vi "Launch.vi"(5 "Sequencer":refnum<class "MessageQ.lvclass">, 6 "State Control":T1, 7 "VolatusAPI":refnum<class "VolatusAPI.lvclass">, 8 "error in (no error)":refnum<class "MultiErrors.lvclass">, 10 "State":T2, 11 "State in":refnum<class "State.lvclass">) -> (0 "error out":refnum<class "MultiErrors.lvclass">, 3 "State out":refnum<class "State.lvclass">)   [LabVIEW 2023, in "VolatusSeq.lvlib" / "State.lvclass"]
uses:
  State.lvclass
  VolatusErrorUtilities/MultiErrors/MultiErrors.lvclass
  VolatusSeqConfig/State.ctl
  VolatusSeqConfig/Step.ctl
  VolatusSeqConfig/Command Config/Command Config.lvclass
  VolatusSeqConfig/Transition Config/Transition Config.lvclass
  VolatusSeqConfig/Debug Flags.ctl
  Volatus/VolatusAPI/VolatusAPI.lvclass
  State Control.ctl
  Sequence Time.ctl
  Variables/Variables.lvclass
  Volatus/MessageQ/MessageQ.lvclass
  lv-promises/Promises/Value/Value.lvclass
  lv-promises/Promises/Promise/Promise.lvclass/Promise.ctl
  lv-promises/Promises/Future/Future.lvclass/Future.ctl
  Loop Async.vi
  lv-promises/Promises/Future/Future.lvclass
  lv-promises/Promises/Promise/Promise.lvclass
  VolatusSeqConfig/VolatusSeqConfig.lvlib
  VolatusSeq.lvlib
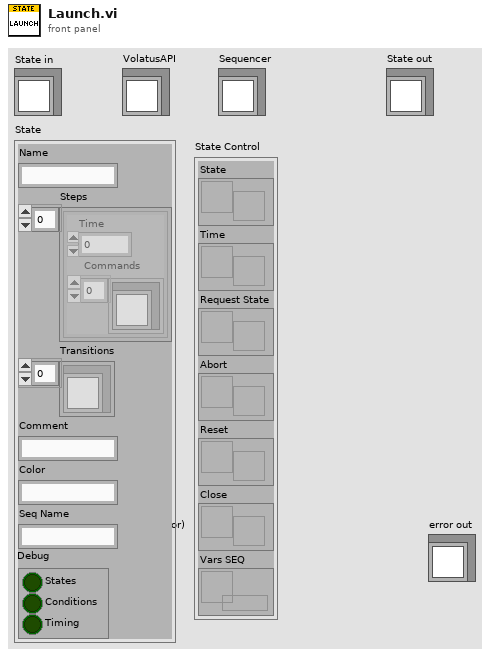
[diagram p1: front panel]
types:
  T1 = typedef "VolatusSeq.lvlib/State Control.ctl" = cluster{"State":refnum<notifier>, "Time":refnum<notifier>, "Request State":refnum<notifier>, "Abort":refnum<notifier>, "Reset":refnum<notifier>, "Close":refnum<notifier>, "Vars SEQ":refnum<queue>}
  T2 = typedef "VolatusSeqConfig.lvlib/State.ctl" = cluster{"Name":string, "Steps":T3[], "Transitions":refnum<class "Transition Config.lvclass">[], "Comment":string, "Color":string, "Seq Name":string, "Debug":T4}
  T3 = typedef "VolatusSeqConfig.lvlib/Step.ctl" = cluster{"Time":dbl, "Commands":refnum<class "Command Config.lvclass">[]}
  T4 = typedef "VolatusSeqConfig.lvlib/Debug Flags.ctl" = cluster{"States":bool, "Conditions":bool, "Timing":bool}
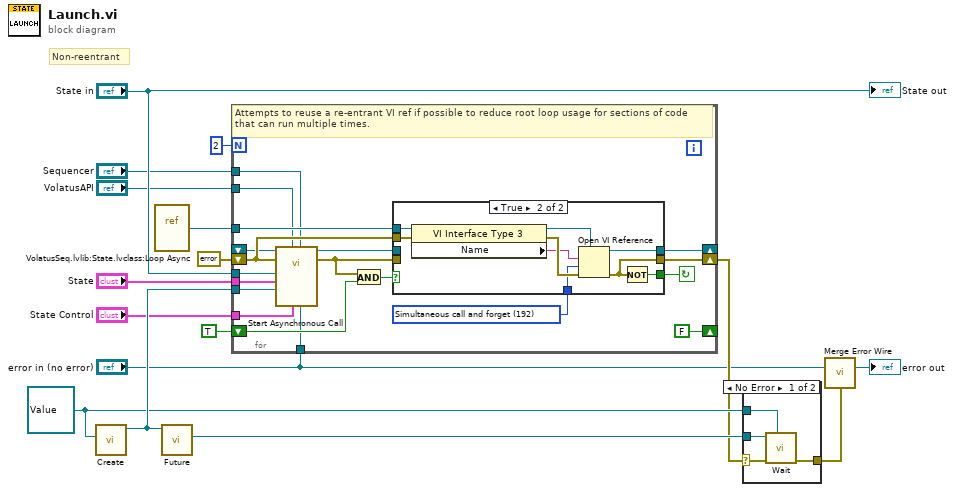
[diagram p0: block diagram]
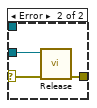
[diagram p3: hidden frame]
diagram:
  w9 = refnum<class "Value.lvclass"> refnum ("Futures:Value.lvclass")
  # "Non-reentrant"
  n1 = call "Create.vi"("Result Type (Variant)"=w9) -> ("Promise"=w11:refnum<class "Promise.lvclass">)  [unwired: 9 in, 1 out]
  n2 = vi-ref "VolatusSeq.lvlib:State.lvclass:Loop Async.vi"() -> (w14:refnum<vi>)
  n3 = call "Future.vi"("Promise in"=w11) -> ("Future"=w10:refnum<class "Future.lvclass">)  [unwired: 9 in, 1 out]
  n4 = for {
    N: 2 -> [_]
    tunnel: w14 -> [w34]
    shift-right: [w33] -> _
    shift-left: _ -> [w32]
    shift-right: [w30] -> w8
    shift-left: errorcluster {"status"=FALSE, "code"=0, "source"=""} ("error constant") -> [w35]
    shift-right: [FALSE] -> _
    shift-left: TRUE -> [w27]
    tunnel: w11 -> [w23]
    tunnel: "State" -> [w22]
    tunnel: "State in" -> [w21]
    tunnel: "VolatusAPI" -> [w20]
    tunnel: "State Control" -> [w19]
    tunnel: "error in (no error)" -> [w18]
    tunnel: "Sequencer" -> [w17]
    stop <- w26 continue-if-true
    w24 = 192 items=["Record modifications"=1, "Open templates for editing"=2, "Prompt user to save"=4, "Prepare for reentrant run"=8, "Prompt to find missing subVIs"=16, "Hide loading dialog box"=32, "Enable simultaneous calls"=64, "Prepare to call and forget"=128, "Simultaneous call and forget"=192, "Prepare to call and collect"=256, "Simultaneous call and collect"=320]
    # "Attempts to reuse a re-entrant VI ref if possible to reduce root loop usage for sections of code that can run multiple times."
    n5 = call-by-ref "Start Asynchronous Call"(reference=w32, error in=w35, "MultiErrors"=w18, "Sequencer"=w17, "Sequence Control"=w19, "VolatusAPI"=w20, "Promise"=w23, "State"=w22, "State in"=w21) -> (reference out=w31:refnum<vi>, error out=w29:errorcluster)  [unwired: 5 in]
    n6 = And(x=w29, y=w27) -> (x .and. y?=w28:bool)
    n7 = case shown="True" w28 {
      tunnel: w34 -> [_ w45]
      tunnel: w24 -> [_ w43]
      tunnel: [w37 w41] -> w33
      tunnel: w31 -> [w37 _]
      tunnel: [w36 w39] -> w30
      tunnel: w29 -> [w36 _]
      tunnel: w35 -> [_ w40]
      tunnel: [_ w38] -> w26
      frame False {
      }
      frame True {
        n8 = property class="VI Interface Type 3"(reference=w45, error in=w40) -> (reference out=w42:refnum<vi>, error out=w46:errorcluster, "Name"=w44:string)
        n9 = Open VI Reference(type specifier VI Refnum (for type only)=w42, vi path=w44, options=w43, error in (no error)=w46) -> (vi reference=w41:refnum<vi>, error out=w39:errorcluster)  [unwired: 2 in]
        n10 = Not(x=w39) -> (.not. x?=w38:bool)
      }
    }
  }
  n11 = case shown="No Error" w8 {
    selector: w8 -> [w48 w51]
    tunnel: w10 -> [w50 w52]
    tunnel: w9 -> [w49 _]
    tunnel: [w47 w51] -> w2
    frame No Error {
      n12 = call "Wait.vi"("Result Type (Variant)"=w49, "error in (no error)"=w48, "Future in"=w50) -> ("error out"=w47:errorcluster)  [unwired: 7 in, 1 out]
    }
    frame Error {
      n13 = call "Release.vi"("Future in"=w52) -> ()  [unwired: 11 in]
    }
  }
  n14 = call "Merge Error Wire.vi"("error in (no error)"=w2, "MultiErrors in"="error in (no error)") -> ("MultiErrors out"=→"error out":refnum<class "MultiErrors.lvclass">)  [unwired: 13 in]
  "State out" <- "State in"
